vi "SetColor.vi"(8 "error in (no error)":errorcluster, 10 "Color":u32(colorbox), 11 "ColorRGB in":refnum<class "ColorRGB.lvclass">) -> (0 "error out":errorcluster, 3 "ColorRGB out":refnum<class "ColorRGB.lvclass">)   [LabVIEW 2021, in "Picture2D.lvlib" / "ColorRGB.lvclass"]
uses:
  ColorRGB.lvclass
  ColorRGB.lvclass/ColorRGB.ctl
  Color/Color.lvclass
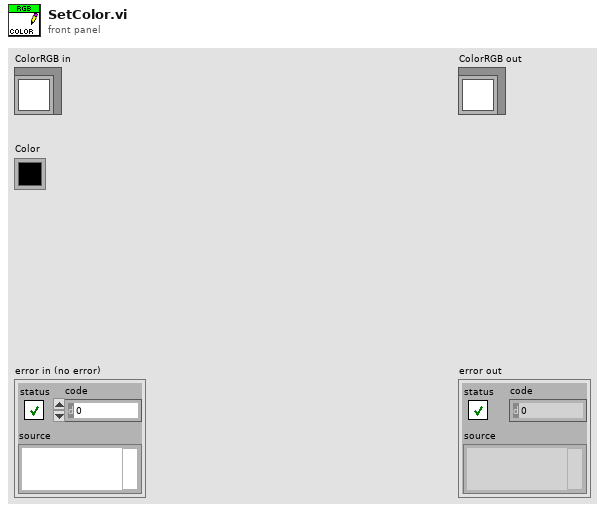
[diagram p1: front panel]
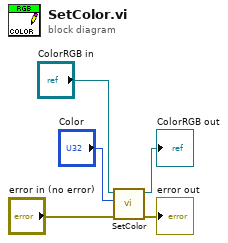
[diagram p0: block diagram]
diagram:
  n1 = call-parent "SetColor.vi"("error in (no error)"="error in (no error)", "Color"="Color", "Color in"="ColorRGB in") -> ("error out"=→"error out":errorcluster, "Color out"=→"ColorRGB out":refnum<class "ColorRGB.lvclass">)  [unwired: 7 in]
